vi "9_nov.vi"() -> ()   [LabVIEW 2020]
uses:
  <instrlib>/Agilent B2900 Series/Public/Configure/Measurement/Configure Measurement (Resistance).vi
  <instrlib>/Agilent B2900 Series/Public/Data/Read Measurement Result (Single Point).vi
  <instrlib>/Agilent B2900 Series/Agilent B2900 Series.lvlib
panel:
  out "Measured Current (A)":dbl
  out "Measured Voltage (Volts)":dbl
  in  "Enable Current Measurement (T: Enable)":bool=TRUE
  in  "Enable Voltage Measurement (T: Enable)":bool=TRUE
  in  "Enable Resistance Measurement (F: Disable)":bool
  in  "SELECT DEVICE":refnum<visa-resource-name>="COM1"
  out "Measured Resistance (ohms)":dbl
  # "MEASURED VALUES"
  # "ENABLE MODES"
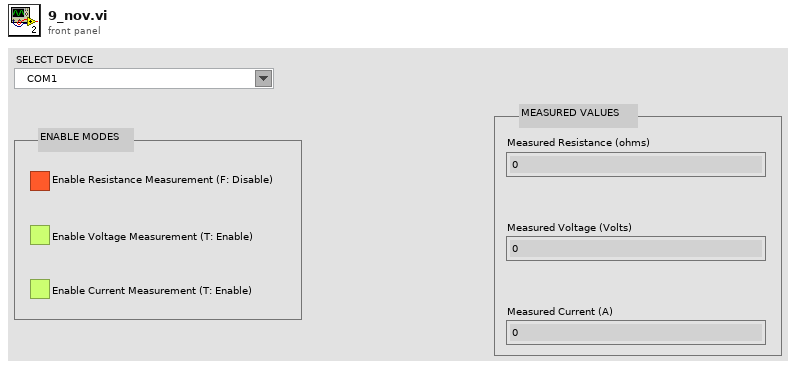
[diagram p1: front panel]
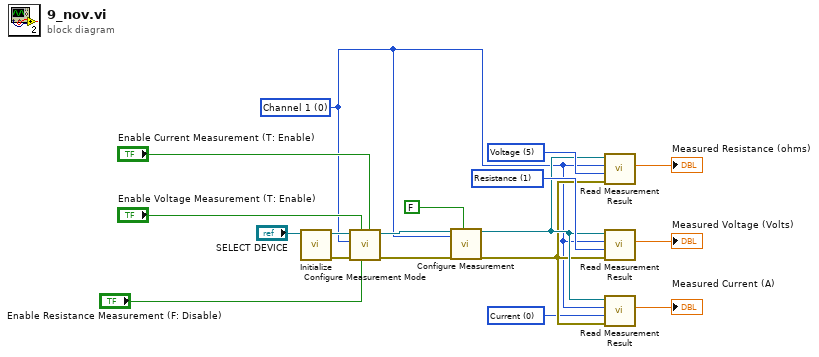
[diagram p0: block diagram]
diagram:
  w3 = 0 items=["Current", "Resistance", "Source Output Setting", "Status", "Time", "Voltage"] ("Data Mode (5: Voltage)")
  w7 = 1 items=["Current", "Resistance", "Source Output Setting", "Status", "Time", "Voltage"] ("Data Mode (5: Voltage)")
  w1 = 0 items=["Channel 1", "Channel 2"] ("Channel (0: Channel 1)")
  w17 = 5 items=["Current", "Resistance", "Source Output Setting", "Status", "Time", "Voltage"] ("Data Mode (5: Voltage)")
  n1 = call <instrlib>:"Initialize.vi"("VISA resource name"="SELECT DEVICE") -> ("error out"=w8:errorcluster, "VISA resource name out"=w9:refnum<visa-resource-name>)  [unwired: 9 in]
  n2 = call <instrlib>:"Configure Measurement Mode.vi"("Enable Current Measurement (T: Enable)"="Enable Current Measurement (T: Enable)", "Enable Resistance Measurement (F: Disable)"="Enable Resistance Measurement (F: Disable)", "Enable Voltage Measurement (T: Enable)"="Enable Voltage Measurement (T: Enable)", "error in (no error)"=w8, "Channel (0: Channel 1)"=w1, "VISA resource name"=w9) -> ("error out"=w15:errorcluster, "VISA resource name out"=w16:refnum<visa-resource-name>)  [unwired: 4 in]
  n3 = call-poly <instrlib>:"Configure Measurement.vi"("VISA resource name"=w16, "Channel (0: Channel 1)"=w1, "error in (no error)"=w15, "Enable Resistance Compensation (F: Disable)"=FALSE) -> ("VISA resource name out"=w5:refnum<visa-resource-name>, "error out"=w4:errorcluster)  [unwired: 14 in]
  n4 = call-poly <instrlib>:"Read Measurement Result.vi"("error in (no error)"=w4, "Data Mode (5: Voltage)"=w17, "Channel (0: Channel 1)"=w1, "VISA resource name"=w5) -> ("Measurement Result"=→"Measured Resistance (ohms)":dbl)  [unwired: 5 in, 2 out]
  n5 = call-poly <instrlib>:"Read Measurement Result.vi"("error in (no error)"=w4, "Data Mode (5: Voltage)"=w7, "Channel (0: Channel 1)"=w1, "VISA resource name"=w5) -> ("Measurement Result"=→"Measured Voltage (Volts)":dbl)  [unwired: 5 in, 2 out]
  n6 = call-poly <instrlib>:"Read Measurement Result.vi"("error in (no error)"=w4, "Data Mode (5: Voltage)"=w3, "Channel (0: Channel 1)"=w1, "VISA resource name"=w5) -> ("Measurement Result"=→"Measured Current (A)":dbl)  [unwired: 5 in, 2 out]
